vi "Fetch SensorID.vi"(8 "error in (no error)":errorcluster, 10 "SQL query":string, 11 "Refnum in":T1) -> (0 "error out":errorcluster, 2 "SensorID":i32, 3 "Refnum out":T1)   [LabVIEW 2026, in "Database.lvlib"]
uses:
  Database.lvlib
  <vilib>/addons/database/Connection.llb/Conn ObjectReference.ctl
  <vilib>/addons/database/Recordset.llb/Rec Fetch Integer Data (R).vi
  <vilib>/addons/database/Recordset.llb/Rec Destroy - Connection.vi
  <vilib>/addons/database/Connection.llb/Conn Execute.vi
  <vilib>/addons/database/NI_Database_API.lvlib
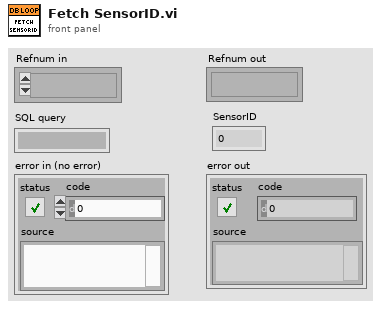
[diagram p1: front panel]
types:
  T1 = typedef "NI_Database_API.lvlib/Conn ObjectReference.ctl" = refnum<k1>
  T2 = typedef "NI_Database_API.lvlib/Rec ObjectReference.ctl" = refnum<k1>
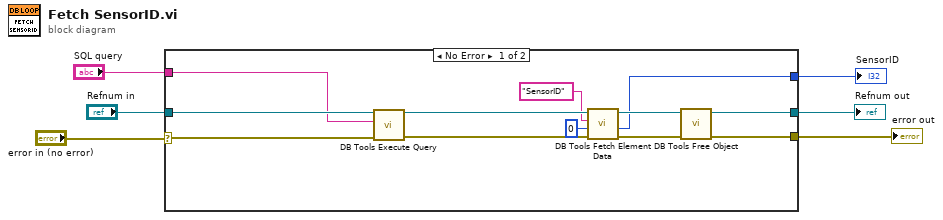
[diagram p0: block diagram]
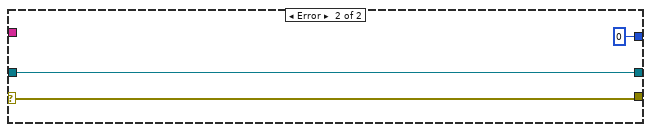
[diagram p2: hidden frame]
diagram:
  n1 = case shown="No Error" "error in (no error)" {
    selector: "error in (no error)" -> [w12 w21]
    tunnel: [w18 w21] -> w6
    tunnel: [w17 w20] -> w5
    tunnel: "Refnum in" -> [w16 w20]
    tunnel: [w13 0 ("data")] -> w4
    tunnel: "SQL query" -> [w7 _]
    frame No Error {
      n2 = call-poly <vilib>:"DB Tools Execute Query.vi"("error in (no error)"=w12, "SQL query"=w7, "connection reference"=w16) -> ("error out"=w8:errorcluster, "recordset reference"=w10:T2)  [unwired: 5 in]
      n3 = call-poly <vilib>:"DB Tools Fetch Element Data.vi"("error in (no error)"=w8, "type"=0, "column index"="SensorID" ("type"), "recordset reference"=w10) -> ("error out"=w15:errorcluster, "data"=w13:i32, "recordset reference out"=w14:T2)  [unwired: 3 in]
      n4 = call-poly <vilib>:"DB Tools Free Object.vi"("error in (no error)"=w15, "recordset reference"=w14) -> ("error out"=w18:errorcluster, "connection reference"=w17:T1)  [unwired: 8 in]
    }
    frame Error {
    }
  }
  "error out" <- w6
  "Refnum out" <- w5
  "SensorID" <- w4
